vi "Create CAL Chunks.vi"(11 "Flash Data Array":u8[](array[numeric])=[21, 178, 54, 1, 68, 65, 84, 65, 95, 83, 69, 84, 0, 0, 5, 172, 0, 3, 0, 104, 48, 48, 48, 52, 86, 87, 51, 55, 49, 45, 48, 77, 69, 95, 75, 0, 0, 0, 0, 0, 86, 87, 51, 55, 49, 32, 74, 101, 116, 116, 97, 44, 32, 73, 110, 97, 108, 102, 97, 0, 0, 0, 0, 0, 0, 0, 0, 0, 0, 0, 0, 0, 0, 0, 0, 0, 0, 0, 0, 0, 0, 0, 0, 0, 0, 0, 0, 0, 0, 115, 113, 11, 55, 51, 55, 49, 48, 66, 86, 87, 51, 55, 49, 48, 72, 69, 78, 68, 2, 21, 61, 83, 247, 139, 193, 236, 172, 85, 14, 71, 200, 114, 223, 179, 250, 0, 0, 0, 0, 0, 58, 152, 0, 0, 0, 50, 15, 160, 50, 200, 0, 130, 0, 1, 70, 80, 25, 100, 46, 224, 31, 64, 78, 32, 26, 244, 0, 40, 1, 244, 0, 200, 0, 25, 0, 25, 0, 150, 0, 150, 1, 244, 1, 244, 0, 2, 0, 2, 0, 255, 0, 254, 0, 100, 0, 0, 0, 10, 0, 50, 0, 100, 0, 220, 0, 253, 0, 2, 0, 2, 0, 6, 0, 10, 0, 80, 0, 100, 0, 0, 0, 50, 0, 100, 0, 0, 0, 50, 0, 100, 0, 80, 0, 80, 50, 200, 3, 182, 0, 100, 254, 112, 0, 230, 0, 250, 4, 176, 7, 8, 74, 56, 5, 220, 7, 208, 108, 205, 7, 208, 27, 88, 7, 208, 96, 0, 32, 0, 33, 52, 1, 144, 0, 172, 1, 144, 1, 144, 93, 192, 0, 50, 0, 27, 5, 86, 3, 232, 1, 59, 5, 79, 0, 176, 0, 176, 0, 176, 0, 27, 3, 232, 0, 8, 50, 200, 0, 220, 0, 10, 0, 72, 27, 88, 0, 80, 5, 173, 35, 40, 9, 196, 74, 56, 66, 104, 0, 210, 62, 128, 6, 64, 26, 244, 29, 76, 3, 232, 33, 52, 2, 0, 0, 0, 0, 0, 0, 0, 5, 0, 0, 10, 15, 110, 228, 0, 1, 2, 3, 4, 0, 1, 2, 3, 4, 0, 1, 2, 3, 4, 6, 24, 10, 32, 28, 127, 126, 2, 1, 0, 10, 2, 1, 3, 1, 2, 2, 2, 2, 3, 40, 8, 0, 100, 0, 0, 0, 0, 0, 0, 0, 0, 0, 0, 0, 0, 4, 4, 20, 90, 20, 128, 255, 240, 255, 63, 255, 135, 7, 192, 0, 43, 2, 161, 0, 0, 0, 1, 87, 192, 0, 50, 0, 30, 255, 226, 2, 188, 0, 27, 5, 173, 0, 240, 0, 30, 0, 30, 1, 144, 1, 144, 4, 176, 0, 166, 3, 132, 0, 230, 0, 240, 1, 59, 1, 244, 1, 244, 1, 244, 5, 25, 236, 239, 140, 5, 130, 140, 5, 130, 9, 9, 170, 0, 0, 0, 0, 1, 87, 192, 0, 50, 0, 40, 255, 216, 2, 188, 0, 30, 3, 132, 0, 240, 0, 50, 0, 50, 1, 144, 1, 144, 2, 88, 0, 200, 1, 144, 0, 198, 0, 200, 0, 200, 3, 132, 1, 244, 1, 244, 5, 25, 236, 239, 120, 5, 110, 100, 5, 90, 9, 9, 170, 0, 0, 0, 1, 173, 89, 199, 132, 164, 244, 175, 60, 253, 33, 53, 140, 72, 106, 195, 65, 0, 0, 54, 0, 34, 55, 80, 0, 0, 0, 0, 0, 0, 0, 0, 20, 5, 128, 0, 0, 70, 0, 55, 50, 100, 0, 0, 0, 0, 0, 0, 0, 0, 252, 0, 0, 0, 0, 70, 0, 18, 50, 50, 0, 0, 0, 0, 0, 200, 0, 254, 0, 50, 0, 0, 0, 70, 0, 18, 50, 50, 0, 0, 0, 0, 0, 120, 0, 254, 0, 70, 0, 0, 1, 44, 0, 230, 50, 50, 0, 0, 0, 0, 0, 200, 0, 254, 75, 0, 0, 0, 1, 104, 0, 220, 90, 130, 0, 0, 0, 0, 0, 0, 0, 0, 0, 5, 0, 0, 0, 72, 0, 34, 80, 130, 0, 0, 0, 0, 0, 0, 0, 0, 32, 8, 128, 0, 0, 130, 0, 72, 90, 130, 0, 0, 0, 0, 0, 0, 0, 0, 2, 0, 0, 0, 0, 0, 0, 0, 50, 50, 0, 0, 0, 0, 0, 0, 0, 0, 0, 0, 0, 0, 0, 0, 0, 0, 50, 50, 0, 0, 0, 0, 0, 0, 0, 0, 0, 0, 0, 0, 0, 96, 0, 52, 50, 100, 0, 0, 0, 0, 0, 0, 0, 0, 0, 252, 0, 0, 2, 208, 2, 58, 0, 50, 0, 0, 0, 0, 0, 0, 0, 0, 0, 15, 0, 0, 0, 140, 0, 100, 0, 50, 0, 0, 0, 0, 0, 0, 0, 0, 0, 18, 0, 0, 4, 76, 2, 208, 0, 50, 0, 0, 0, 0, 0, 0, 0, 0, 251, 0, 0, 0, 1, 44, 0, 230, 50, 50, 0, 0, 0, 0, 0, 120, 0, 254, 0, 70, 0, 0, 1, 44, 0, 230, 50, 50, 0, 0, 0, 0, 0, 180, 0, 254, 23, 50, 0, 0, 40, 0, 0, 35, 4, 176, 1, 14, 1, 14, 0, 20, 0, 0, 0, 0, 21, 85, 0, 35, 23, 32, 0, 60, 21, 32, 0, 70, 0, 0, 0, 70, 0, 0, 0, 70, 0, 0, 0, 200, 5, 20, 0, 35, 0, 176, 117, 48, 0, 100, 0, 0, 0, 0, 0, 70, 0, 0, 0, 70, 0, 0, 0, 70, 0, 0, 0, 70, 0, 0, 0, 70, 0, 0, 62, 128, 42, 248, 255, 190, 1, 72, 11, 184, 5, 20, 0, 176, 0, 176, 0, 50, 0, 0, 50, 200, 3, 32, 3, 32, 1, 64, 0, 100, 0, 0, 0, 60, 0, 120, 1, 144, 0, 0, 0, 0, 255, 0, 0, 0, 0, 0, 255, 0, 0, 0, 0, 0, 255, 0, 128, 0, 62, 128, 12, 205, 23, 112, 243, 51, 0, 6, 0, 3, 3, 232, 0, 125, 0, 50, 0, 50, 0, 88, 0, 100, 2, 0, 0, 128, 14, 16, 12, 128, 62, 128, 1, 4, 1, 1, 4, 2, 2, 2, 3, 8, 8, 4, 1, 4, 7, 20, 0, 0, 20, 255, 2, 20, 0, 34, 253, 40, 20, 200, 40, 27, 0, 0, 20, 50, 30, 6, 0, 20, 50, 19, 50, 95, 5, 50, 100, 20, 6, 20, 5, 60, 32, 0, 85, 50, 25, 30, 200, 100, 40, 55, 1, 55, 255, 2, 3, 100, 100, 2, 1, 200, 0, 10, 20, 12, 100, 1, 100, 1, 9, 4, 4, 4, 4, 40, 0, 8, 0, 0, 30, 40, 4, 5, 2, 5, 5, 1, 1, 3, 0, 1, 2, 1, 5, 1, 0, 4, 1, 5, 100, 55, 55, 255, 255, 32, 30, 1, 5, 20, 1, 144, 110, 0, 32, 2, 135, 40, 1, 6, 6, 2, 78, 54, 224, 0, 0, 0, 0, 0, 0, 0, 0, 0, 0, 20, 0, 0, 0, 0, 21, 80, 0, 70, 0, 0, 0, 70, 0, 0, 0, 70, 0, 0, 0, 70, 0, 0, 0, 70, 0, 0, 0, 0, 0, 0, 0, 0, 0, 0, 117, 48, 0, 100, 0, 0, 0, 0, 0, 70, 0, 0, 0, 70, 0, 0, 0, 70, 0, 0, 0, 70, 0, 0, 0, 70, 0, 0, 62, 128, 42, 248, 255, 190, 1, 72, 11, 184, 0, 0, 0, 0, 0, 0, 0, 0, 0, 0, 50, 200, 3, 32, 3, 32, 0, 0, 0, 100, 0, 0, 0, 60, 0, 120, 1, 144, 0, 0, 0, 0, 255, 0, 0, 0, 0, 0, 255, 0, 0, 0, 0, 0, 255, 0, 128, 0, 62, 128, 12, 205, 23, 112, 243, 51, 0, 0, 0, 0, 11, 184, 0, 125, 0, 50, 0, 50, 0, 125, 0, 100, 2, 0, 0, 128, 14, 16, 12, 128, 62, 128, 1, 4, 1, 1, 4, 2, 3, 3, 3, 8, 8, 4, 1, 4, 7, 20, 0, 0, 20, 255, 2, 20, 0, 34, 253, 40, 20, 200, 6, 0, 0, 0, 0, 0, 0, 6, 0, 60, 60, 0, 0, 95, 5, 50, 255, 20, 8, 8, 0, 0, 0, 8, 80, 60, 30, 30, 0, 0, 10, 10, 1, 55, 255, 255, 1, 80, 80, 255, 2, 200, 0, 10, 20, 15, 251, 4, 251, 4, 9, 4, 4, 4, 4, 40, 0, 8, 0, 0, 30, 40, 4, 5, 2, 5, 5, 1, 1, 3, 0, 1, 2, 1, 5, 1, 0, 4, 1, 5, 100, 255, 255, 255, 255, 0, 30, 1, 5, 30, 1, 116, 75, 0, 40, 2, 135, 45, 1, 10, 6, 2, 72, 54, 128, 0, 0, 0, 0, 0, 12, 144, 49, 221, 68, 65, 84, 65, 95, 69, 78, 68, 255, 255, 255, 255] format="%.0x") -> (3 "Array 2":u8[][](array[numeric]) format="%.0x")   [LabVIEW 2018]
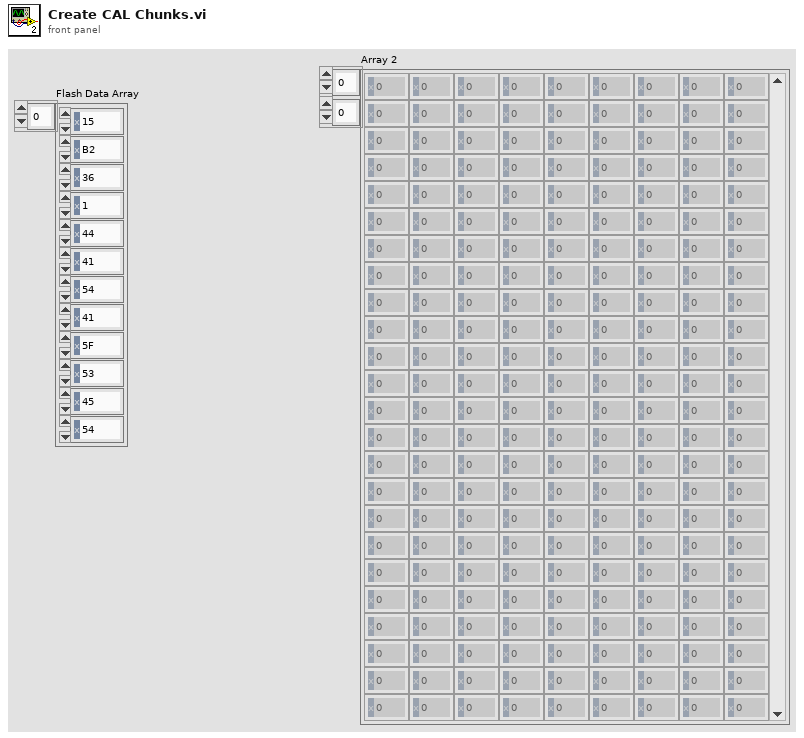
[diagram p1: front panel]
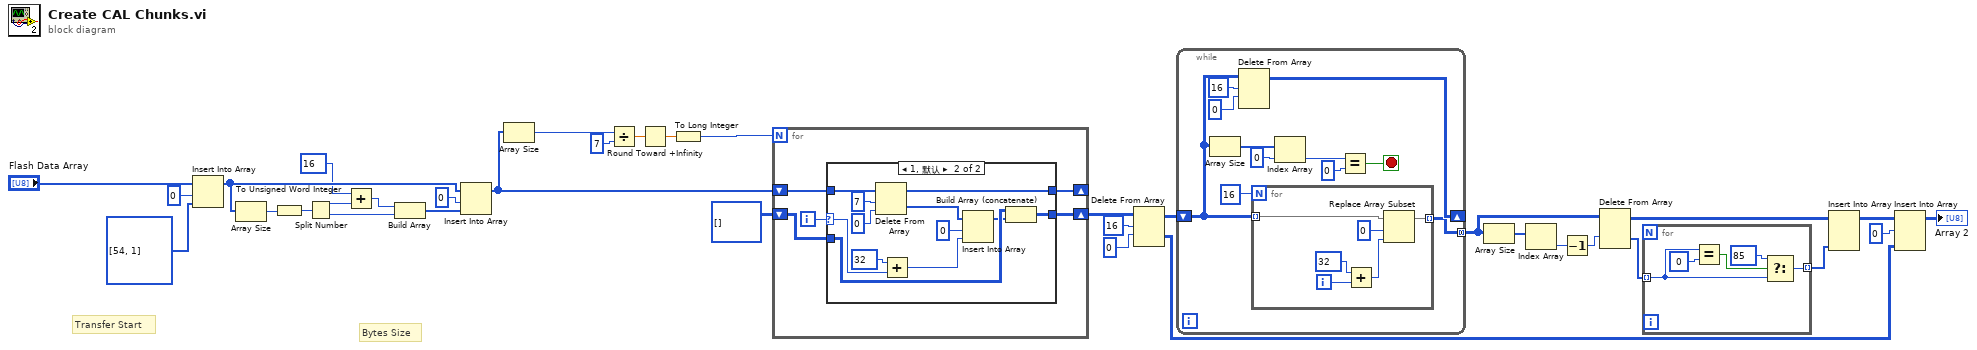
[diagram p0: block diagram]
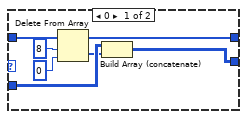
[diagram p2: hidden frame]
diagram:
  # "Bytes Size"
  # "Transfer Start"
  n1 = Insert Into Array(array="Flash Data Array", index=0, new element=u8[] [54, 1] ("Flash Data Array")) -> (w7:u8[])
  n2 = Array Size(array=w7) -> (size(s)=w10:i32)
  n3 = To Unsigned Word Integer(number=w10) -> (unsigned 16bit integer=w12:u16)
  n4 = Split Number(x=w12) -> (hi(x)=w2:u8, lo(x)=w11:u8)
  n5 = Add(x=u8 16 ("hi"), y=w2) -> (x+y=w1:u8)
  n6 = Build Array(w1, w11) -> (w5:u8[])
  n7 = Insert Into Array(array=w7, index=0, new element=w5) -> (w4:u8[])
  n8 = Array Size(array=w4) -> (size(s)=w34:i32)
  n9 = Divide(x=w34, y=7) -> (x/y=w31:dbl)
  n10 = Round Toward +Infinity(x=w31) -> (ceil(x): smallest int >= x=w30:dbl)
  n11 = To Long Integer(number=w30) -> (32bit integer=w32:i32)
  n12 = for {
    N: w32 -> [_]
    shift-right: [w36] -> w26
    shift-left: u8[][] [] ("Array") -> [w37]
    shift-right: [w35] -> _
    shift-left: w4 -> [w38]
    i -> [w39]
    n13 = case shown="1, 默认" w39 {
      selector: w39 -> [_ w47]
      tunnel: w38 -> [w46 w58]
      tunnel: w37 -> [w45 w57]
      tunnel: [w44 w53] -> w36
      tunnel: [w40 w49] -> w35
      frame 0 {
        n14 = Delete From Array(array=w46, length=8, index=0) -> (deleted portion=w41:u8[], array with subset deleted=w40:u8[])
        n15 = Build Array (concatenate)(w45, w41) -> (w44:u8[][])
      }
      frame 1, Default {
        n16 = Delete From Array(array=w58, length=7, index=0) -> (deleted portion=w48:u8[], array with subset deleted=w49:u8[])
        n17 = Add(x=u8 32 ("new element/subarray"), y=w47) -> (x+y=w51:i32)
        n18 = Insert Into Array(array=w48, index=0, new element=w51) -> (w54:u8[])
        n19 = Build Array (concatenate)(w57, w54) -> (w53:u8[][])
      }
    }
  }
  n20 = Delete From Array(array=w26, length=16, index (row)=0) -> (deleted portion=w24:u8[][], array with subset deleted=w25:u8[][])  [unwired: 1 in]
  n21 = while {
    shift-right: [w61] -> _
    shift-left: w25 -> [w60]
    tunnel: [w59] -> w17 mode=concatenating
    stop <- w66 stop-if-true
    n22 = Array Size(array=w60) -> (size(s)=w68:i32[])
    n23 = Delete From Array(array=w60, length=16, index (row)=0) -> (array with subset deleted=w61:u8[][])  [unwired: 1 in, 1 out]
    n24 = for {
      N: 16 -> [_]
      tunnel: [w71] -> w59 mode=indexing
      tunnel: w60 -> [w70] mode=indexing
      i -> [w73]
      n25 = Add(x=u8 32 ("new element/subarray"), y=w73) -> (x+y=w72:i32)
      n26 = Replace Array Subset(array=w70, new element=w72, index=0) -> (w71:u8[])
    }
    n27 = Index Array(array=w68, index=0) -> (element=w67:i32)
    n28 = Equal?(x=w67, y=0) -> (x = y?=w66:bool)
  }
  n29 = Array Size(array=w17) -> (size(s)=w22:i32[])
  n30 = Index Array(array=w22) -> (element=w21:i32)  [unwired: 1 in]
  n31 = Decrement(x=w21) -> (x-1=w18:i32)
  n32 = Delete From Array(array=w17, index (row)=w18) -> (deleted portion=w19:u8[], array with subset deleted=w14:u8[][])  [unwired: 2 in]
  n33 = for {
    tunnel: w19 -> [w78] mode=indexing
    tunnel: [w76] -> w16 mode=indexing
    n34 = Equal?(x=w78, y=u8 0) -> (x = y?=w79:bool)
    n35 = Select(t=u8 85, s=w79, f=w78) -> (s? t:f=w76:u8)
  }
  n36 = Insert Into Array(array=w14, new element=w16) -> (w15:u8[][])  [unwired: 2 in]
  n37 = Insert Into Array(array=w15, index (row)=0, new element=w24) -> (→"Array 2":u8[][])  [unwired: 1 in]
